vi "set_additional_soft_limit.vi"(8 "error in (no error)":errorcluster caption="错误输入（无错误）", 10 "additional soft limit":T1(array[cluster]), 11 "MotorSystem输入":refnum<class "MotorSystem.lvclass">) -> (0 "error out":errorcluster caption="错误输出", 3 "MotorSystem输出":refnum<class "MotorSystem.lvclass">)   [LabVIEW 2016, in "MotionControl.lvlib" / "MotorSystem.lvclass"]
uses:
  <userlib>/MotionControl/MotorSystem/MotorSystem.lvclass
  <userlib>/MotionControl/MotorSystem/MotorSystem.lvclass/MotorSystem.ctl
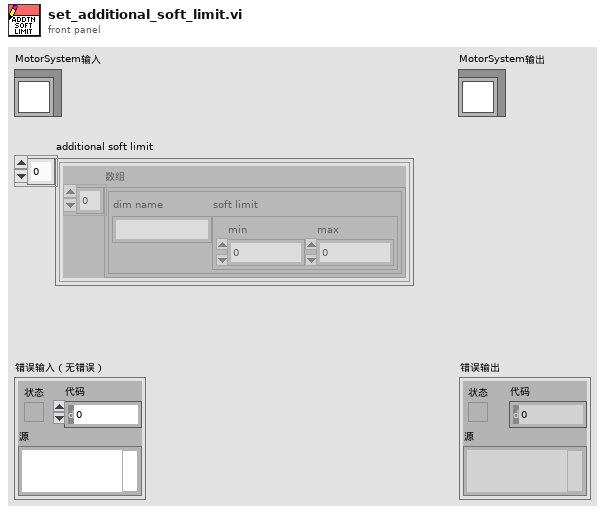
[diagram p1: front panel]
types:
  T1 = cluster{"数组":cluster{"dim name":string, "soft limit":cluster{"min":dbl, "max":dbl}}[]}[]
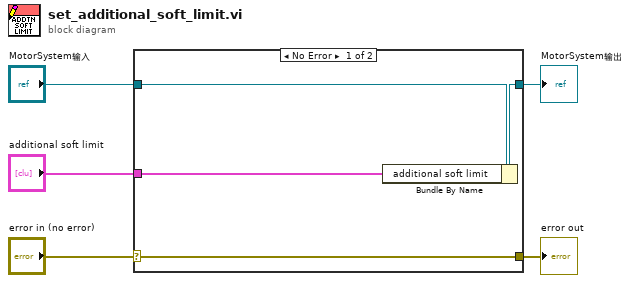
[diagram p0: block diagram]
diagram:
  n1 = case shown="No Error" "error in (no error)" {
    selector: "error in (no error)" -> [w9 w10]
    tunnel: [w9 w10] -> w4
    tunnel: [w7 w11] -> w2
    tunnel: "MotorSystem输入" -> [w8 w11]
    tunnel: "additional soft limit" -> [w6 _]
    frame No Error {
      n2 = Bundle By Name(cluster=w8, "additional soft limit"=w6) -> (w7:refnum<class "MotorSystem.lvclass">)
    }
    frame Error {
    }
  }
  "error out" <- w4
  "MotorSystem输出" <- w2
